vi "LJM_eAddresses.vi"(0 "Handle In":i32, 1 "NumFrames":i32=-1, 5 "aAddresses":i32[](array[numeric]), 7 "aTypes":i32[](array[numeric]), 9 "aValuesIn":dbl[](array[numeric]) format="%.2f", 11 "error in":errorcluster, 12 "aWrites":i32[](array[ring]) items=["Read", "Write"], 13 "aNumValues":i32[](array[numeric])) -> (4 "Handle Out":i32, 10 "aValuesOut":dbl[](array[numeric]) format="%.2f", 14 "ErrorAddress":i32, 15 "error out":errorcluster)   [LabVIEW 2020]
uses:
  Library/Frameworks/LabJackM.framework
panel:
  # "This function does not check or modify the aValuesIn array.  You must initialize it properly.  We recommend\nalways using eAddresses2D in LabVIEW rather than eAddresses."
  # "1/20/2015:  Default value of NumFrames changed to -1.  If\nNumFrames = -1, then the NumFrames control is ignored\nand the size of aNames/aAddresses is used to determine how\nmany frames there are."
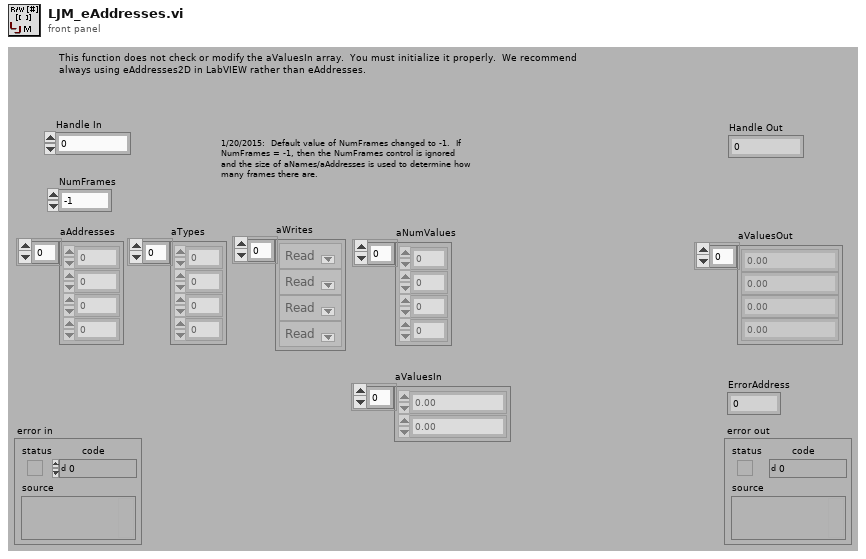
[diagram p1: front panel]
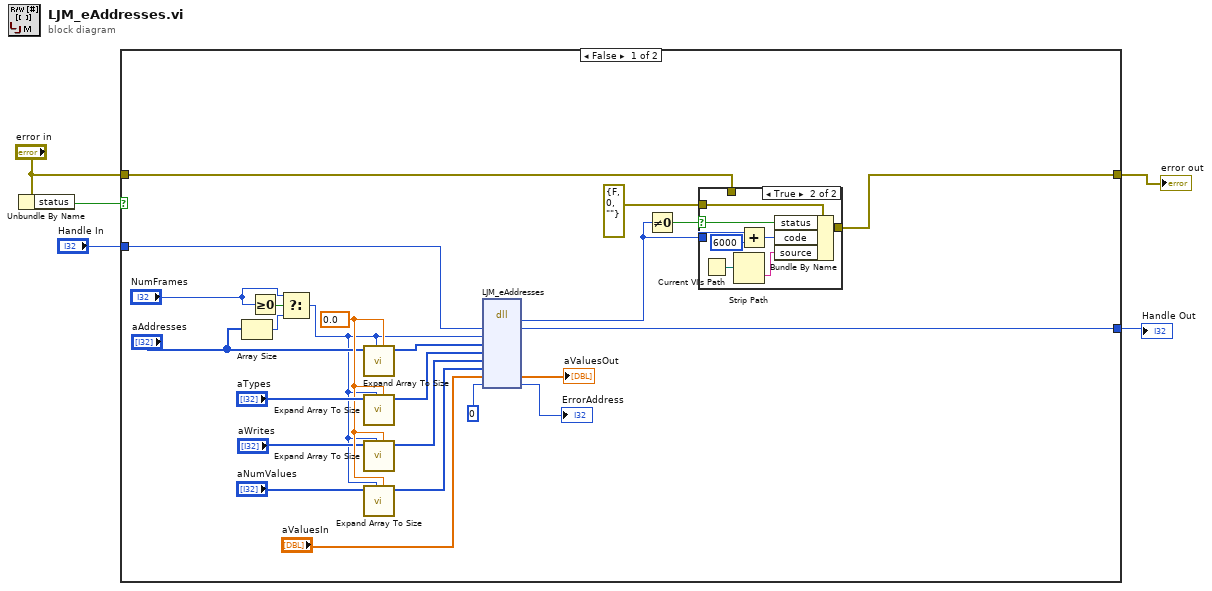
[diagram p0: block diagram]
diagram:
  n1 = Unbundle By Name("error in") -> ("status"=w5:bool)
  n2 = case shown="False" w5 {
    tunnel: "error in" -> [w26 w40]
    tunnel: [w25 w40] -> w3
    tunnel: [w13 w39] -> w2
    tunnel: "Handle In" -> [w12 w39]
    frame False {
      w21 = 0.0 ("Default Value")
      n3 = Array Size(array="aAddresses") -> (size(s)=w10:i32)
      n4 = Greater Or Equal To 0?(x="NumFrames") -> (x >= 0?=w9:bool)
      n5 = Select(t="NumFrames", s=w9, f=w10) -> (s? t:f=w6:i32)
      n6 = call "Expand Array To Size.vi"("Default Value"=w21, "# Elements"=w6, "I32 Array In"="aAddresses") -> ("I32 Array Out"=w24:i32[])  [unwired: 4 in, 4 out]
      n7 = call "Expand Array To Size.vi"("Default Value"=w21, "# Elements"=w6, "I32 Array In"="aTypes") -> ("I32 Array Out"=w22:i32[])  [unwired: 4 in, 4 out]
      n8 = call "Expand Array To Size.vi"("Default Value"=w21, "# Elements"=w6, "I32 Array In"="aWrites") -> ("I32 Array Out"=w18:i32[])  [unwired: 4 in, 4 out]
      n9 = call "Expand Array To Size.vi"("Default Value"=w21, "# Elements"=w6, "I32 Array In"="aNumValues") -> ("I32 Array Out"=w17:i32[])  [unwired: 4 in, 4 out]
      n10 = dll-call lib="Library/Frameworks/LabJackM.framework" fn="LJM_eAddresses"("Handle"=w12, "NumFrames"=w6, "aAddresses"=w24, "aTypes"=w22, "aWrites"=w18, "aNumValues"=w17, "aValues"="aValuesIn", "ErrorFrame"=u32 0) -> ("return type"=w29:i32, "Handle"=w13:i32, "aValues"=→"aValuesOut":dbl[], "ErrorFrame"=→"ErrorAddress":i32)  [unwired: 8 in, 2 out]
      n11 = Not Equal To 0?(x=w29) -> (x != 0?=w28:bool)
      n12 = case shown="True" w28 {
        selector: w28 -> [_ w37]
        tunnel: [w30 w38] -> w25
        tunnel: errorcluster {"status"=FALSE, "code"=0, "source"=""} ("error IO") -> [_ w36]
        tunnel: w29 -> [_ w32]
        tunnel: w26 -> [w30 _]
        frame False {
        }
        frame True {
          n13 = Current VI's Path() -> (path=w34:path)
          n14 = Strip Path(path=w34) -> (name=w35:string)  [unwired: 1 out]
          n15 = Add(x=w32, y=6000) -> (x+y=w33:i32)
          n16 = Bundle By Name(cluster=w36, "status"=w37, "code"=w33, "source"=w35) -> (w38:errorcluster)
        }
      }
    }
    frame True {
    }
  }
  "error out" <- w3
  "Handle Out" <- w2
